vi "Part 2.vi"(11 "Input":string="46threevqs8114\nthreetwoonez1gtrd\n6ffxbtff\n769twotwo6rv9\ngjrcjrkvghthreegqqrg82qbct\nzkxjhgprtrlcfeight795five8\n99seven3vdcgvmvxtjtwodc5\nthree5eightthree3four3vtkkqrgxs\nfour863mrrnrsxrkone\nsevenntgvnrrqfvxh2ttnkgffour8fiveone\n49fbsfb\n3rbmlsksg\nztgszqjjsrtmgqx6572\n3bqnfxkdbonesixseven\nmfgx32ftpbhgngm7\nfzrpfhbfvj6dbxbtfs7twofksfbshrzkdeightwoqg\n2xcftwo\ncshmmltsml4fiveeightdn\neightthsix1\ntwo1gvfxcqnrfnbeightthreexznhbmmk\n3917sevenvxqxntcgxskh\nksctcnfxdsk96drlbjkthreesfqlvnpvfbcbmg\n8nvrmzfs46\n5dbgltmgg1xvtqfkdxsrxzltwo1pgqlqndlc\neight7four6rpbtmjzj5\n41seven\ngpmfhninexxgqr6\n15sixdrhxzcmqf\n8fivettgmcs...") -> (3 "Output":i64)   [LabVIEW 2021]
uses:
  <userlib>/_OpenG.lib/string/string.llb/Convert EOLs (String)__ogtk.vi
panel:
  # "54251"
  # "54217"
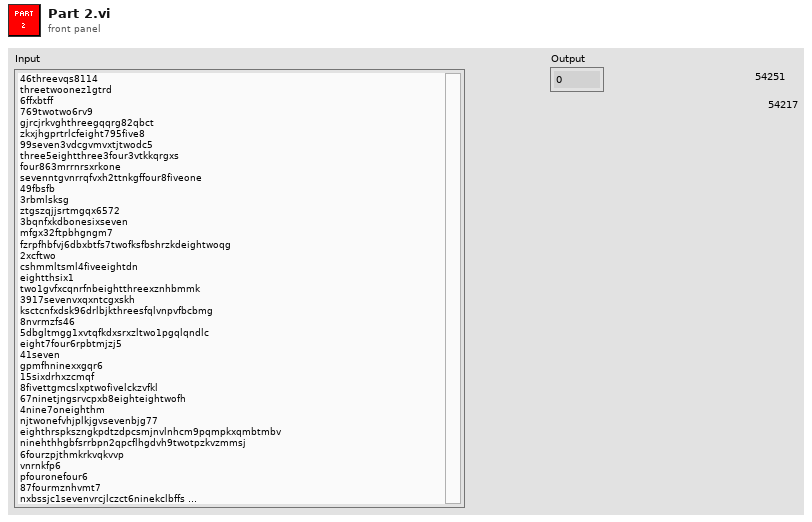
[diagram p1: front panel]
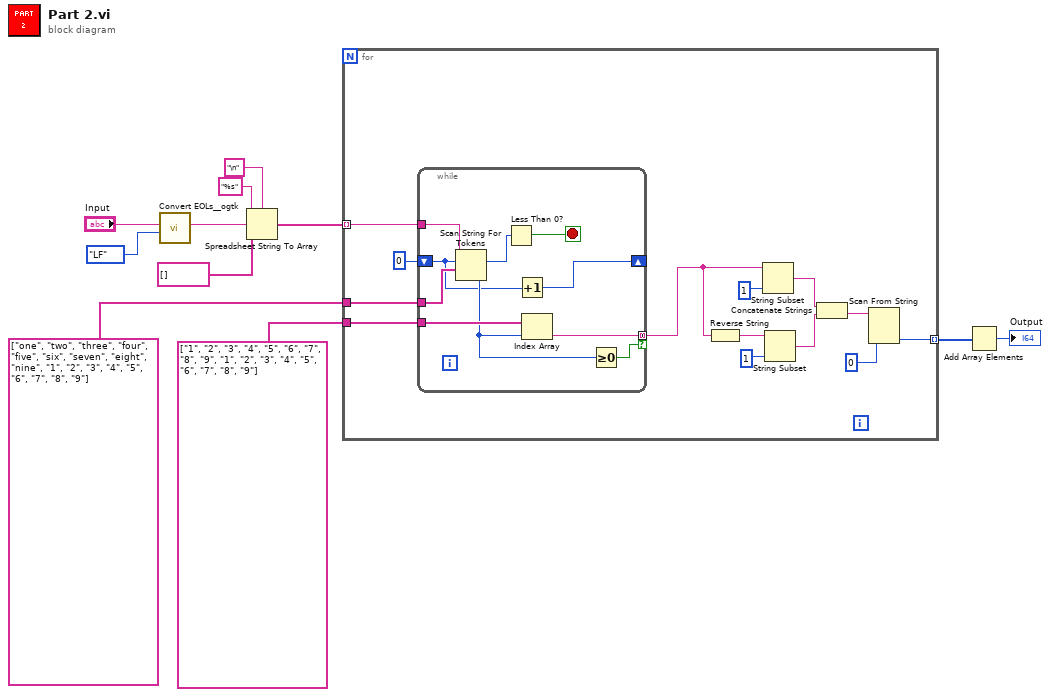
[diagram p0: block diagram]
diagram:
  n1 = call-poly <userlib>:"Convert EOLs__ogtk.vi"("Convert to:"=enum16{"CR", "LF", "CRLF"}."LF", "String in"="Input") -> ("String out"=w7:string)  [unwired: 9 in]
  n2 = Spreadsheet String To Array(delimiter (Tab)="\n", format string="%s", spreadsheet string=w7, array type (2D Dbl)=string[] []) -> (array=w5:string[])
  n3 = for {
    tunnel: w5 -> [w16] mode=indexing
    tunnel: [w23] -> w4 mode=indexing
    tunnel: string[] ["one", "two", "three", "four", "five", "six", "seven", "eight", "nine", "1", "2", "3", "4", "5", "6", "7", "8", "9"] -> [w18]
    tunnel: string[] ["1", "2", "3", "4", "5", "6", "7", "8", "9", "1", "2", "3", "4", "5", "6", "7", "8", "9"] -> [w17]
    n4 = while {
      tunnel: w18 -> [w30]
      tunnel: w17 -> [w34]
      shift-right: [w25] -> _
      shift-left: 0 -> [w26]
      tunnel: [w32] -> w12 mode=concatenating if=w28
      tunnel: w16 -> [w31]
      stop <- w33 stop-if-true
      n5 = Scan String For Tokens(7:w30, 8:w26, 9:w31) -> (0:w29:i32, 2:w27:i32)  [unwired: 3 in, 2 out]
      n6 = Less Than 0?(x=w27) -> (x < 0?=w33:bool)
      n7 = Increment(x=w26) -> (x+1=w25:i32)
      n8 = Index Array(array=w34, index=w29) -> (element=w32:string)
      n9 = Greater Or Equal To 0?(x=w29) -> (x >= 0?=w28:bool)
    }
    n10 = Reverse String(1:w12) -> (0:w21:string)
    n11 = String Subset(string=w12, length (rest)=1) -> (substring=w20:string)  [unwired: 1 in]
    n12 = String Subset(string=w21, length (rest)=1) -> (substring=w19:string)  [unwired: 1 in]
    n13 = Concatenate Strings(w20, w19) -> (w24:string)
    n14 = Scan From String(input string=w24, default 1=i64 0 ("Output")) -> (output 1=w23:i64)  [unwired: 3 in, 3 out]
  }
  n15 = Add Array Elements(numeric array=w4) -> (sum=→"Output":i64)
